vi "Write NET_HttpRequestMessage.vi"(8 "error in (no error)":errorcluster, 10 "NET_HttpRequestMessage":refnum<k24>, 11 "HttpRequestMessage in":refnum<class "HttpRequestMessage.lvclass">) -> (0 "error out":errorcluster, 3 "HttpRequestMessage out":refnum<class "HttpRequestMessage.lvclass">)   [LabVIEW 2018, in "LabVIEWHTTPClient_NET.lvlib" / "HttpRequestMessage.lvclass"]
uses:
  HttpRequestMessage.lvclass
  System.Net.Http
  HttpRequestMessage.lvclass/HttpRequestMessage.ctl
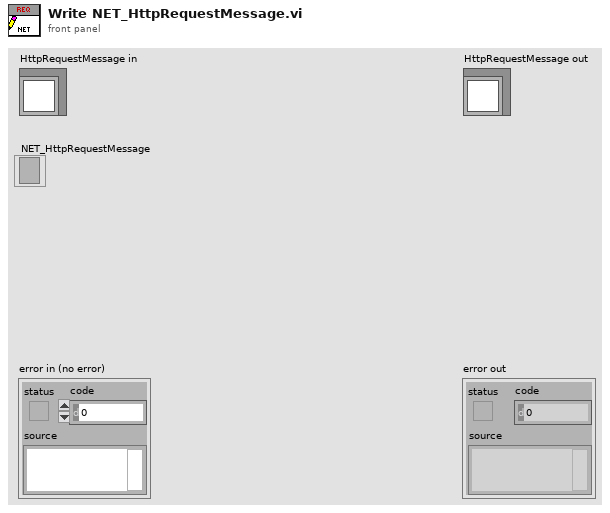
[diagram p1: front panel]
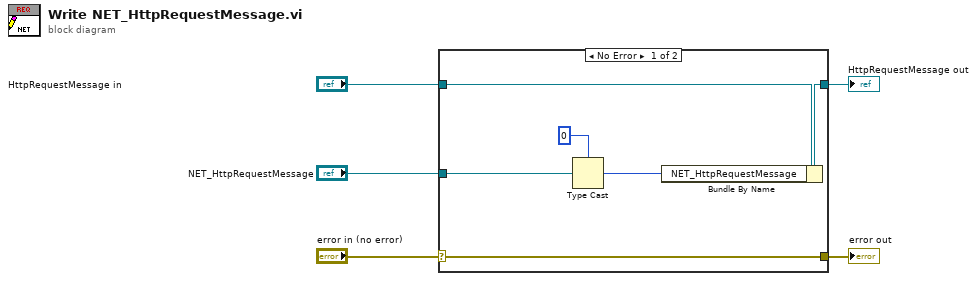
[diagram p0: block diagram]
diagram:
  n1 = case shown="No Error" "error in (no error)" {
    selector: "error in (no error)" -> [w11 w12]
    tunnel: [w11 w12] -> w4
    tunnel: [w9 w13] -> w2
    tunnel: "HttpRequestMessage in" -> [w10 w13]
    tunnel: "NET_HttpRequestMessage" -> [w8 _]
    frame No Error {
      n2 = Type Cast(type=i64 0 ("NET_HttpRequestMessage"), x=w8) -> (*(type *) &x=w6:i64)
      n3 = Bundle By Name(cluster=w10, "NET_HttpRequestMessage"=w6) -> (w9:refnum<class "HttpRequestMessage.lvclass">)
    }
    frame Error {
    }
  }
  "error out" <- w4
  "HttpRequestMessage out" <- w2
